vi "Static Error Handling.To String.Integer.Decimal.I8 v2.vi"(1 "value":i8) -> (0 "value as string":string)   [LabVIEW 2016]
doc: "Converts the provided <B>value</B> into a decimal-formatted string."
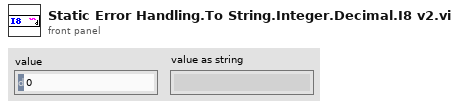
[diagram p1: front panel]
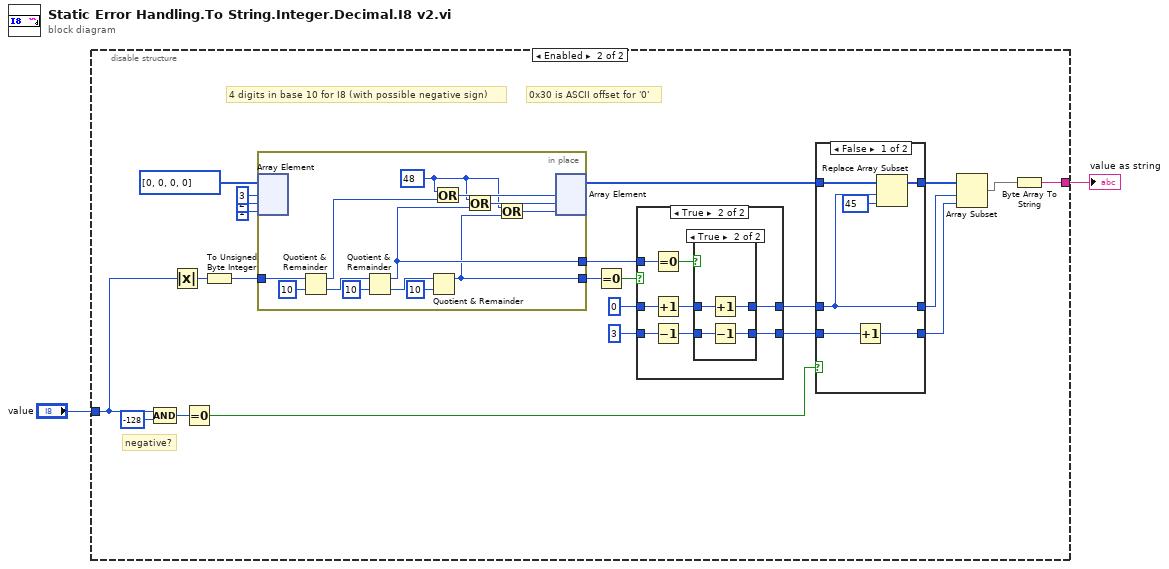
[diagram p0: block diagram]
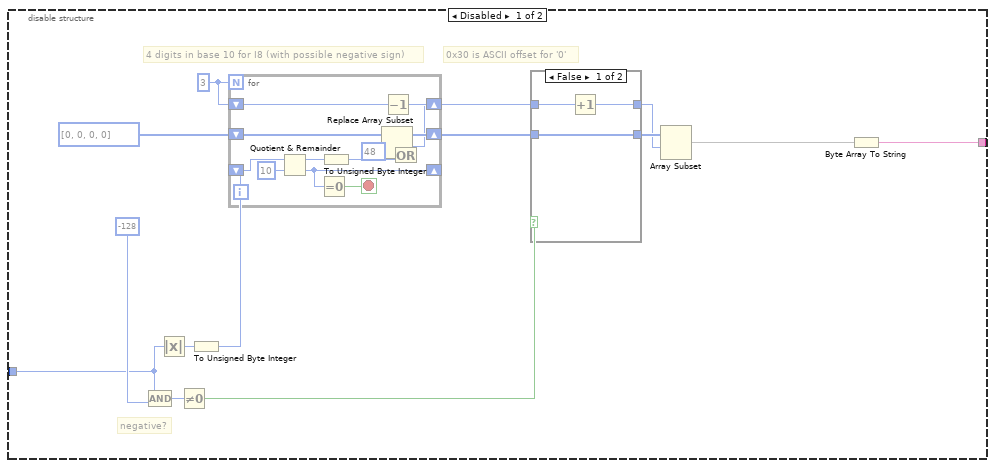
[diagram p2: hidden frame]
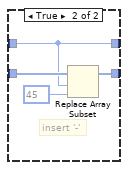
[diagram p3: hidden frame]
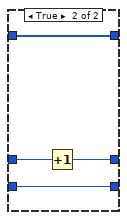
[diagram p4: hidden frame]
diagram:
  n1 = disable-structure shown="Enabled" {
    disable-tunnel: [w16 w38] -> w2
    disable-tunnel: "value" -> [w3 w54]
    frame Disabled {
      w11 = 3
      # "negative?"
      # "0x30 is ASCII offset for '0'"
      # "4 digits in base 10 for I8 (with possible negative sign)"
      n2 = Compound Arithmetic op=AND(w3, i8 -128 ("y")) -> (w10:i8)
      n3 = Absolute Value(x=w3) -> (abs(x)=w4:i8)
      n4 = Not Equal To 0?(x=w10) -> (x != 0?=w9:bool)
      n5 = To Unsigned Byte Integer(number=w4) -> (unsigned 8bit integer=w13:u8)
      n6 = for {
        N: w11 -> [_]
        shift-right: [w27] -> w12
        shift-left: u8[] [0, 0, 0, 0] -> [w21]
        shift-right: [w23] -> _
        shift-left: w13 -> [w18]
        shift-right: [w20] -> w8
        shift-left: w11 -> [w19]
        stop <- w17 stop-if-true
        n7 = Quotient & Remainder(x=w18, y=u8 10) -> (x-y*floor(x/y)=w24:u8, floor(x/y)=w23:u8)
        n8 = Equal To 0?(x=w23) -> (x = 0?=w17:bool)
        n9 = To Unsigned Byte Integer(number=w24) -> (unsigned 8bit integer=w22:u8)
        n10 = Decrement(x=w19) -> (x-1=w20:i32)
        n11 = Or(x=u8 48 ("y"), y=w22) -> (x .or. y?=w28:u8)
        n12 = Replace Array Subset(array=w21, new element=w28, index=w19) -> (w27:u8[])
      }
      n13 = case shown="False" w9 {
        tunnel: w12 -> [w31 w35]
        tunnel: w8 -> [w30 w32]
        tunnel: [w31 w33] -> w7
        tunnel: [w29 w32] -> w5
        frame False {
          n14 = Increment(x=w30) -> (x+1=w29:i32)
        }
        frame True {
          # "insert '-'"
          n15 = Replace Array Subset(array=w35, new element=u8 45 ("y"), index=w32) -> (w33:u8[])
        }
      }
      n16 = Array Subset(array=w7, index=w5) -> (w6:u8[])  [unwired: 1 in]
      n17 = Byte Array To String(unsigned byte array=w6) -> (string=w16:string)
    }
    frame Enabled {
      # "negative?"
      # "0x30 is ASCII offset for '0'"
      # "4 digits in base 10 for I8 (with possible negative sign)"
      n18 = Compound Arithmetic op=AND(w54, i8 -128 ("y")) -> (w57:i8)
      n19 = Absolute Value(x=w54) -> (abs(x)=w55:i8)
      n20 = Equal To 0?(x=w57) -> (x = 0?=w45:bool)
      n21 = To Unsigned Byte Integer(number=w55) -> (unsigned 8bit integer=w53:u8)
      n22 = in-place {
        in-place-border: w53 -> [w79]
        in-place-border: [w74] -> w52
        in-place-border: [w75] -> w47
        w69 = u8 48 ("y")
        n23 = in-place-array #1(u8[] [0, 0, 0, 0], 3, 2, 1) -> ()  [unwired: 3 out]
        n24 = Quotient & Remainder(x=w79, y=u8 10) -> (x-y*floor(x/y)=w73:u8, floor(x/y)=w76:u8)
        n25 = Quotient & Remainder(x=w76, y=u8 10) -> (x-y*floor(x/y)=w75:u8, floor(x/y)=w77:u8)
        n26 = Quotient & Remainder(x=w77, y=u8 10) -> (x-y*floor(x/y)=w74:u8)  [unwired: 1 out]
        n27 = Or(x=w69, y=w73) -> (x .or. y?=w72:u8)
        n28 = Or(x=w69, y=w75) -> (x .or. y?=w71:u8)
        n29 = Or(x=w69, y=w74) -> (x .or. y?=w70:u8)
        n30 = in-place-array #1(w72, w71, w70) -> (w44:u8[])  [unwired: 3 out]
      }
      n31 = Equal To 0?(x=w52) -> (x = 0?=w51:bool)
      n32 = case shown="True" w51 {
        tunnel: u8 0 ("index") -> [w83 w89]
        tunnel: u8 3 ("index") -> [w82 w86]
        tunnel: [w83 w85] -> w46
        tunnel: [w82 w84] -> w43
        tunnel: w47 -> [_ w90]
        frame False {
        }
        frame True {
          n33 = Equal To 0?(x=w90) -> (x = 0?=w91:bool)
          n34 = Increment(x=w89) -> (x+1=w87:u8)
          n35 = Decrement(x=w86) -> (x-1=w88:u8)
          n36 = case shown="True" w91 {
            tunnel: w87 -> [w93 w97]
            tunnel: w88 -> [w92 w96]
            tunnel: [w93 w95] -> w85
            tunnel: [w92 w94] -> w84
            frame False {
            }
            frame True {
              n37 = Increment(x=w97) -> (x+1=w95:u8)
              n38 = Decrement(x=w96) -> (x-1=w94:u8)
            }
          }
        }
      }
      n39 = case shown="False" w45 {
        tunnel: w46 -> [w61 w68]
        tunnel: [w61 w67] -> w41
        tunnel: w44 -> [w63 w66]
        tunnel: w43 -> [w60 w65]
        tunnel: [w62 w66] -> w42
        tunnel: [w59 w65] -> w40
        frame False {
          n40 = Increment(x=w60) -> (x+1=w59:u8)
          n41 = Replace Array Subset(array=w63, new element=u8 45 ("y"), index=w61) -> (w62:u8[])
        }
        frame True {
          n42 = Increment(x=w68) -> (x+1=w67:u8)
        }
      }
      n43 = Array Subset(array=w42, index=w41, length=w40) -> (w39:u8[])
      n44 = Byte Array To String(unsigned byte array=w39) -> (string=w38:string)
    }
  }
  "value as string" <- w2
